vi "init stage.vi"(8 "error in":errorcluster, 10 "stage motion":T1=enum."fast", 11 "Actuator cluster in":T2={"Actuator COM"="COM14", "Actuator type"=enum."Scientifica"}) -> (0 "error out":errorcluster, 2 "initialization error":bool, 3 "Actuator cluster out":T2={"Actuator COM"="COM14", "Actuator type"=enum."Scientifica"})   [LabVIEW 2015]
uses:
  pipette cleaning/pressure box/cleaning_soft/controls/actuator_type.ctl
  pipette cleaning/pressure box/cleaning_soft/controls/actuator_cluster.ctl
  controls/scope_motion.ctl
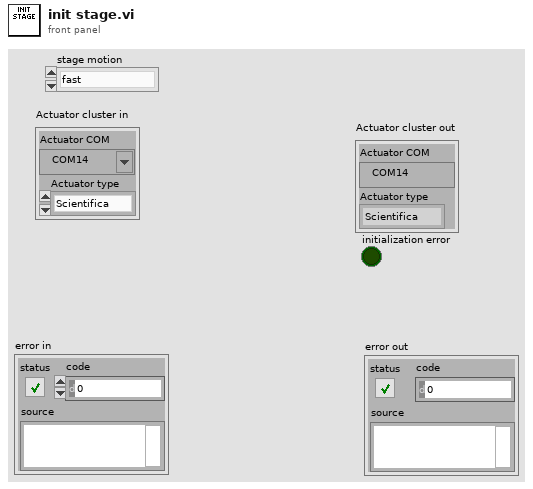
[diagram p1: front panel]
types:
  T1 = typedef "scope_motion.ctl" = enum16{"superSlow", "fast", "slow", "find slice speed", "slow_dualPatch"}
  T2 = typedef "actuator_cluster.ctl" = cluster{"Actuator COM":refnum<visa-resource-name>, "Actuator type":T3}
  T3 = typedef "actuator_type.ctl" = enum16{"Scientifica", "Sutter", "Demo", "Off"}
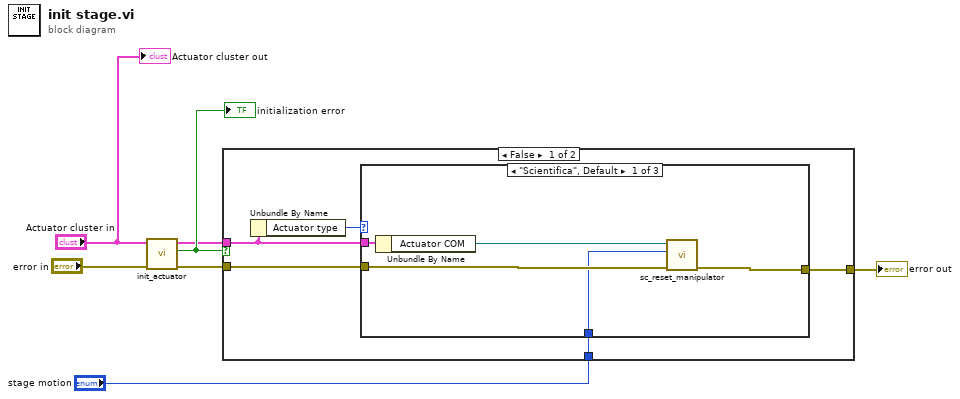
[diagram p0: block diagram]
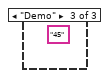
[diagram p3: hidden frame]
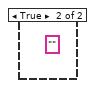
[diagram p4: hidden frame]
diagram:
  n1 = call "init_actuator.vi"("error in"="error in", "Actuator cluster in"="Actuator cluster in") -> ("error out"=w4:errorcluster, "initialization error"=w6:bool, "Actuator cluster out"=w5:T2)  [unwired: 7 in]
  "initialization error" <- w6
  n2 = case shown="False" w6 {
    tunnel: w5 -> [w11 _]
    tunnel: w4 -> [w10 _]
    tunnel: [w9 _] -> w2
    tunnel: "stage motion" -> [w8 _]
    frame False {
      n3 = Unbundle By Name(w11) -> ("Actuator type"=w12:T3)
      n4 = case shown="\"Scientifica\", Default" w12 {
        tunnel: w11 -> [w17 _ _]
        tunnel: w10 -> [w14 _ _]
        tunnel: [w16 _ _] -> w9
        tunnel: w8 -> [w13 _ _]
        frame "Scientifica", Default {
          n5 = Unbundle By Name(w17) -> ("Actuator COM"=w15:refnum<visa-resource-name>)
          n6 = call "sc_reset_manipulator.vi"("error in (no error)"=w14, "motion"=w13, "visa in"=w15) -> ("error out"=w16:errorcluster)  [unwired: 7 in, 1 out]
        }
        frame "Sutter" {
        }
        frame "Demo" {
          (unwired) "45" ("Response")
        }
      }
    }
    frame True {
      (unwired) "" ("Response")
    }
  }
  "error out" <- w2
  "Actuator cluster out" <- "Actuator cluster in"
